vi "WhirlpoolsExperimentRoshansEdit.vi"(9 "Start sweeping":bool) -> ()   [LabVIEW 2013]
panel:
  out "Experiment ends at:":string
  in  "error in (no error)":errorcluster
  in  "Optional custom folder":string
  out "Sweep":i16
  out "Array":dbl[](array[numeric])
  in  "Step (V)":dbl=0.01 min=-4.0 max=4.0 step=1.0 format="%#.4g"
  out "minutes":dbl caption="Last full sweep took:" format="%#.1g"
  in  "Faster":dbl=10.0
  in  "HigherRate to V1?":bool
  out "Hours":dbl format="%.1f"
  out "Of":i16
  out "Estimated time of experiment:":i16
  in  "Sweeps at each Bias:":i16=1 min=-4 max=4 step=1
  in  "Final Bias (V)":dbl=0.01 min=-4.0 max=4.0 step=0.1 format="%.4f"
  in  "Initial Bias (V)":dbl min=-4.0 max=4.0 step=0.1 format="%.4f"
  in  "V2:":dbl=1.0 min=-4.0 max=4.0 step=0.1 format="%.3f"
  in  "Sweep rate , V/min":dbl=0.6 min=0.0 max=1.0 step=0.01 format="%.5f"
  in  "V1:":dbl min=-4.0 max=4.0 step=0.1 format="%.3f"
  # "Define interval of gate voltage\nfor main Keithley 2400 (address 12):"
  # "Set bias voltages at which sweeps\nare made:"
  # "SourceMeter (address 13)"
  # "min."
  # "= approx."
  # "hours"
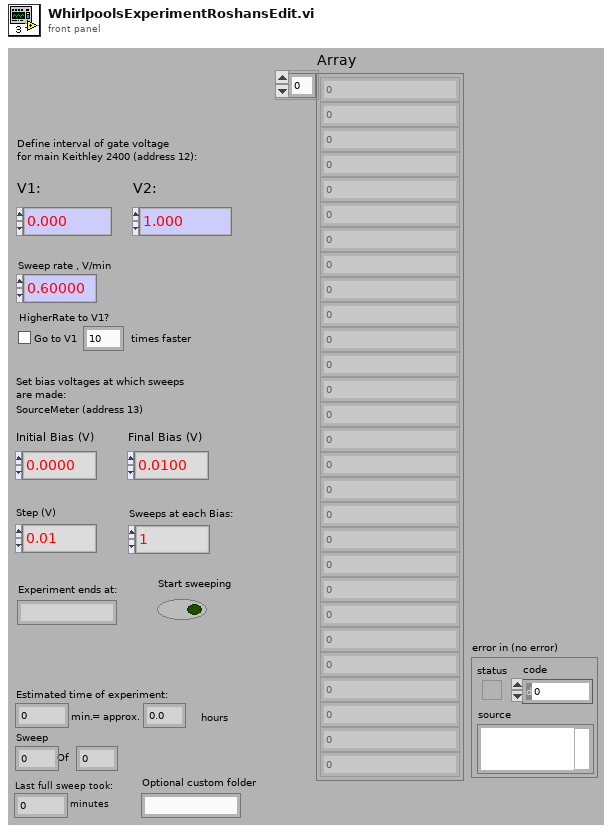
[diagram p1: front panel]
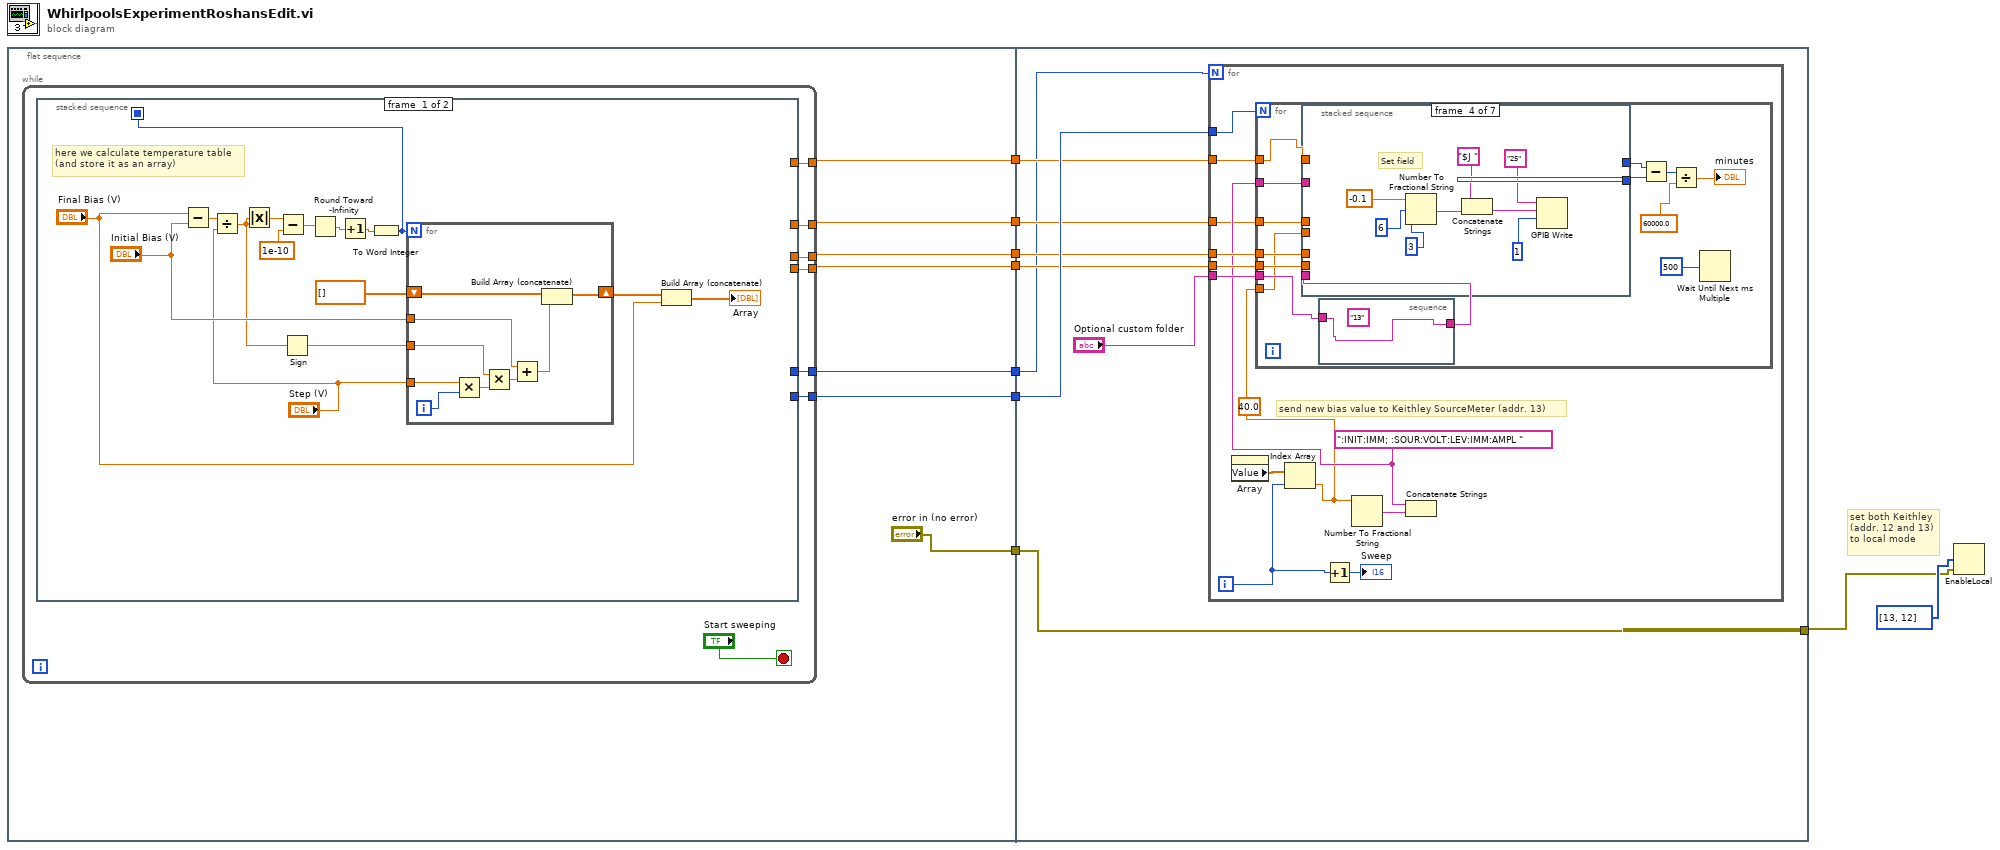
[diagram p0: block diagram]
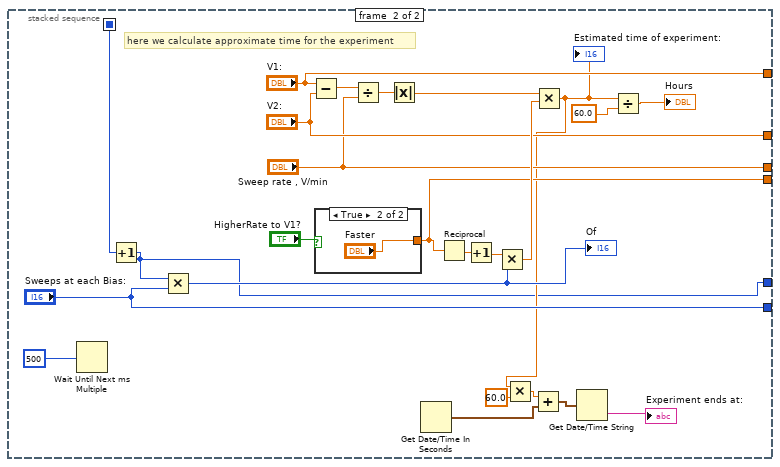
[diagram p2: hidden frame]
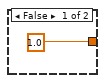
[diagram p3: hidden frame]
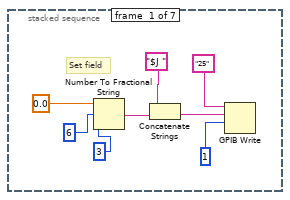
[diagram p4: hidden frame]
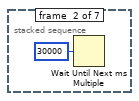
[diagram p5: hidden frame]
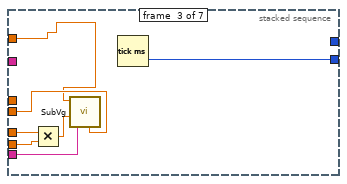
[diagram p6: hidden frame]
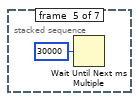
[diagram p7: hidden frame]
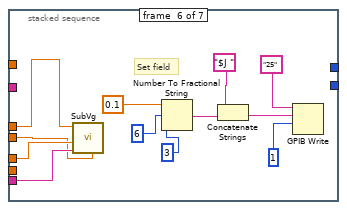
[diagram p8: hidden frame]
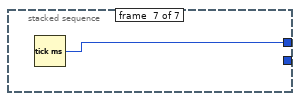
[diagram p9: hidden frame]
diagram:
  # "set both Keithley\n(addr. 12 and 13)\nto local mode"
  n1 = flat-sequence {
    tunnel: [w16] -> w9
    tunnel: [w15] -> w8
    tunnel: [w14] -> w7
    tunnel: [w13] -> w6
    tunnel: [w12] -> w5
    tunnel: [w11] -> w4
    tunnel: ["error in (no error)"] -> w3
    tunnel: w9 -> [w81]
    tunnel: w8 -> [w80]
    tunnel: w7 -> [w79]
    tunnel: w6 -> [w78]
    tunnel: w5 -> [w77]
    tunnel: w4 -> [w76]
    tunnel: w3 -> [w74]
    tunnel: [w74] -> w1
    frame #0 {
      n2 = while {
        tunnel: [w22] -> w16
        tunnel: [w21] -> w15
        tunnel: [w20] -> w14
        tunnel: [w19] -> w13
        tunnel: [w18] -> w12
        tunnel: [w17] -> w11
        stop <- "Start sweeping" stop-if-true
        n3 = stacked-sequence {
          seq-local: [w24 _] -> [_ w56]
          tunnel: [_ "Sweeps at each Bias:"] -> w22
          tunnel: [_ "V1:"] -> w21
          tunnel: [_ "V2:"] -> w20
          tunnel: [_ "Sweep rate , V/min"] -> w19
          tunnel: [_ w57] -> w18
          tunnel: [_ w48] -> w17
          frame #0 {
            # "here we calculate temperature table\n(and store it as an array)"
            n4 = Subtract(x="Final Bias (V)", y="Initial Bias (V)") -> (x-y=w28:dbl)
            n5 = Divide(x=w28, y="Step (V)") -> (x/y=w27:dbl)
            n6 = Absolute Value(x=w27) -> (abs(x)=w37:dbl)
            n7 = Subtract(x=w37, y=1e-10) -> (x-y=w35:dbl)
            n8 = Sign(1:w27) -> (0:w34:dbl)
            n9 = Round Toward -Infinity(1:w35) -> (0:w29:dbl)
            n10 = Increment(x=w29) -> (x+1=w25:dbl)
            n11 = To Word Integer(number=w25) -> (16bit integer=w24:i16)
            n12 = for {
              N: w24 -> [_]
              shift-right: [w39] -> w32
              shift-left: dbl[] [] -> [w47]
              tunnel: "Step (V)" -> [w45]
              tunnel: w34 -> [w43]
              tunnel: "Initial Bias (V)" -> [w41]
              i -> [w44]
              n13 = Multiply(x=w45, y=w44) -> (x*y=w46:dbl)
              n14 = Multiply(x=w43, y=w46) -> (x*y=w42:dbl)
              n15 = Add(x=w41, y=w42) -> (x+y=w40:dbl)
              n16 = Build Array (concatenate)(w47, w40) -> (w39:dbl[])
            }
            n17 = Build Array (concatenate)(w32, "Final Bias (V)") -> (→"Array":dbl[])
          }
          frame #1 {
            # "here we calculate approximate time for the experiment"
            n18 = Wait Until Next ms Multiple(millisecond multiple=500) -> ()  [unwired: 1 out]
            n19 = Increment(x=w56) -> (x+1=w48:i16)
            n20 = Multiply(x=w48, y="Sweeps at each Bias:") -> (x*y=w55:i16)
            "Of" <- w55
            n21 = Subtract(x="V1:", y="V2:") -> (x-y=w71:dbl)
            n22 = case shown="True" "HigherRate to V1?" {
              tunnel: [1.0 "Faster"] -> w57
              frame False {
              }
              frame True {
              }
            }
            n23 = Divide(x=w71, y="Sweep rate , V/min") -> (x/y=w70:dbl)
            n24 = Absolute Value(x=w70) -> (abs(x)=w69:dbl)
            n25 = Get Date/Time In Seconds() -> (seconds since 1Jan1904=w52:timestamp)
            n26 = Reciprocal(x=w57) -> (1/x=w59:dbl)
            n27 = Increment(x=w59) -> (x+1=w63:dbl)
            n28 = Multiply(x=w63, y=w55) -> (x*y=w65:dbl)
            n29 = Multiply(x=w69, y=w65) -> (x*y=w49:dbl)
            "Estimated time of experiment:" <- w49
            n30 = Multiply(x=w49, y=60.0) -> (x*y=w53:dbl)
            n31 = Add(x=w53, y=w52) -> (x+y=w51:timestamp)
            n32 = Get Date/Time String(seconds (now)=w51) -> (time string=→"Experiment ends at:":string)  [unwired: 2 in, 1 out]
            n33 = Divide(x=w49, y=60.0) -> (x/y=→"Hours":dbl)
          }
        }
      }
    }
    frame #1 {
      n34 = for {
        N: w76 -> [_]
        tunnel: w81 -> [w92]
        tunnel: w80 -> [w83]
        tunnel: w79 -> [w82]
        tunnel: w78 -> [w91]
        tunnel: w77 -> [w90]
        tunnel: "Optional custom folder" -> [w87]
        i -> [w88]
        (unwired) 40.0
        w85 = ":INIT:IMM; :SOUR:VOLT:LEV:IMM:AMPL " ("data")
        # "send new bias value to Keithley SourceMeter (addr. 13)"
        n35 = property on="Array" class="Arr (strict)"() -> ("Value"=w93:dbl[])  [unwired: 2 in, 2 out]
        n36 = Index Array(array=w93, index=w88) -> (element=w84:dbl)
        n37 = for {
          N: w92 -> [_]
          tunnel: w83 -> [w95]
          tunnel: w82 -> [w94]
          tunnel: w91 -> [w107]
          tunnel: w90 -> [w106]
          tunnel: w87 -> [w99]
          tunnel: w85 -> [w97]
          tunnel: w84 -> [w96]
          n38 = stacked-sequence {
            tunnel: w99 -> [w108]
            tunnel: [w108] -> w98
            frame #0 {
              (unwired) "13"
            }
          }
          n39 = stacked-sequence {
            tunnel: w94 -> [_ _ _ _ _ w142 _]
            tunnel: w107 -> [_ _ w124 _ _ w145 _]
            tunnel: w95 -> [_ _ w118 _ _ _ _]
            tunnel: w106 -> [_ _ w123 _ _ _ _]
            tunnel: [_ _ w121 _ _ _ _] -> w102
            tunnel: [_ _ _ _ _ _ w146] -> w101
            tunnel: w98 -> [_ _ w120 _ _ w144 _]
            tunnel: w97 -> [_ _ _ _ _ _ _]
            tunnel: w96 -> [_ _ w119 _ _ w143 _]
            frame #0 {
              # "Set field"
              n40 = Number To Fractional String(number=0.0, width (-)=6, precision (6)=3) -> (F-format string=w114:string)  [unwired: 1 in]
              n41 = Concatenate Strings("$J ", w114) -> (w113:string)
              n42 = GPIB Write(0:"25", 1:w113, 2:1) -> ()  [unwired: 2 in, 2 out]
            }
            frame #1 {
              n43 = Wait Until Next ms Multiple(millisecond multiple=30000) -> ()  [unwired: 1 out]
            }
            frame #2 {
              n44 = Multiply(x=w124, y=w123) -> (x*y=w122:dbl)
              n45 = call "SubVg.vi"("Target Voltage, V"=w118, "Sweep rate, V/min"=w122, "Custom Folder"=w120, "optional Bias (V)"=w119) -> ()  [unwired: 6 in]
              n46 = Tick Count (ms)() -> (millisecond timer value=w121:u32)
            }
            frame #3 {
              # "Set field"
              n47 = Number To Fractional String(number=-0.1, width (-)=6, precision (6)=3) -> (F-format string=w130:string)  [unwired: 1 in]
              n48 = Concatenate Strings("$J ", w130) -> (w129:string)
              n49 = GPIB Write(0:"25", 1:w129, 2:1) -> ()  [unwired: 2 in, 2 out]
            }
            frame #4 {
              n50 = Wait Until Next ms Multiple(millisecond multiple=30000) -> ()  [unwired: 1 out]
            }
            frame #5 {
              # "Set field"
              n51 = call "SubVg.vi"("Target Voltage, V"=w142, "Sweep rate, V/min"=w145, "Custom Folder"=w144, "optional Bias (V)"=w143) -> ()  [unwired: 6 in]
              n52 = Number To Fractional String(number=0.1, width (-)=6, precision (6)=3) -> (F-format string=w139:string)  [unwired: 1 in]
              n53 = Concatenate Strings("$J ", w139) -> (w138:string)
              n54 = GPIB Write(0:"25", 1:w138, 2:1) -> ()  [unwired: 2 in, 2 out]
            }
            frame #6 {
              n55 = Tick Count (ms)() -> (millisecond timer value=w146:u32)
            }
          }
          n56 = Subtract(x=w101, y=w102) -> (x-y=w105:u32)
          n57 = Divide(x=w105, y=60000.0) -> (x/y=→"minutes":dbl)
          n58 = Wait Until Next ms Multiple(millisecond multiple=500) -> ()  [unwired: 1 out]
        }
        n59 = Increment(x=w88) -> (x+1=→"Sweep":i32)
        n60 = Number To Fractional String(number=w84) -> (F-format string=w86:string)  [unwired: 3 in]
        n61 = Concatenate Strings(w85, w86) -> ()  [unwired: 1 out]
      }
    }
  }
  n62 = EnableLocal(2:w1, 3:i32[] [13, 12]) -> ()  [unwired: 1 in, 2 out]
